vi "LVClass_WavefrontCorrector dtor.vi"(0 "WavefrontCorrector in":refnum<class "WavefrontCorrector.lvclass">, 11 "error in (no error)":errorcluster) -> (4 "WavefrontCorrector out":refnum<class "WavefrontCorrector.lvclass">, 15 "error out":errorcluster)   [LabVIEW 2020, in "WavefrontCorrector.lvclass"]
doc: "WavefrontCorrector destructor.\n\n--------------------------------------------------------------------------------\n\n<B>correctorIn </B> : WavefrontCorrector object.\n<B>correctorOut </B> : WavefrontCorrector object.\n<B>ErrorIn </B> : Error\n<B>ErrorOut </B> : Error\n\n--------------------------------------------------------------------------------"
uses:
  WavefrontCorrector.lvclass
  Controls/Wavefront Corrector states - ONE.ctl
  WavefrontCorrector.lvclass/WavefrontCorrector.ctl
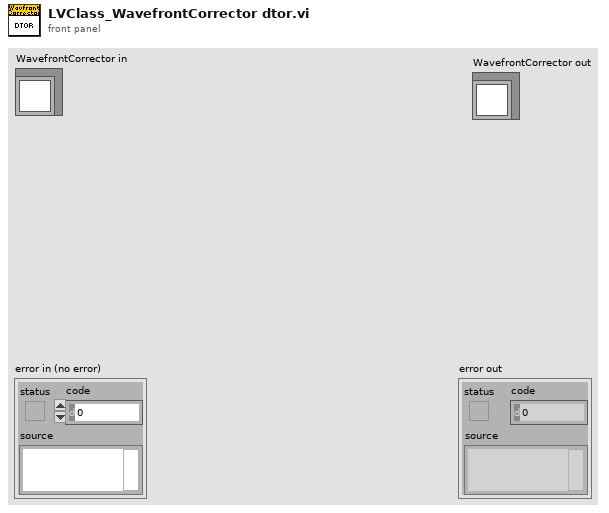
[diagram p1: front panel]
types:
  T1 = typedef "Wavefront Corrector states - ONE.ctl" = cluster{"Max":sgl, "Min":sgl, "Validity":enum16{"valid", "fixed", "invalid"}, "Fixed_Position":sgl}
  T2 = cluster{"Sleep after command apply_ms":i32, "Wavefront Corrector State":T1[]}
  T3 = typedef "Handle creation.ctl" = enum16{"By ctor", "By write function"}
  T4 = typedef "ClassID.ctl" = i64
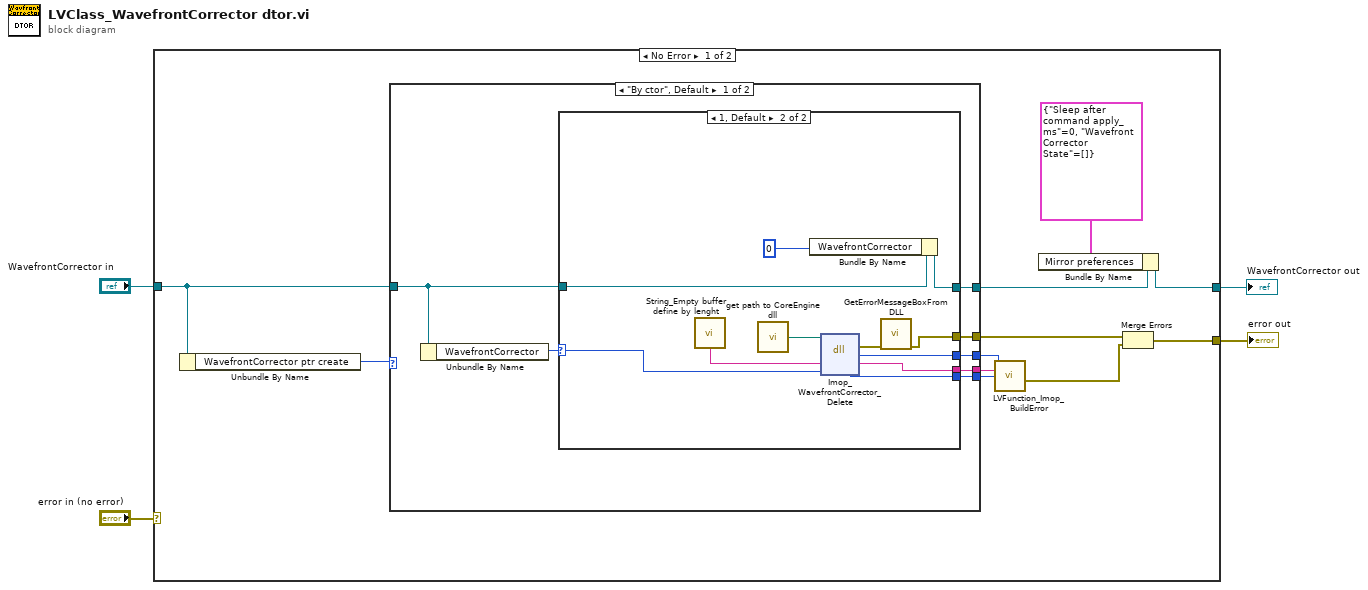
[diagram p0: block diagram]
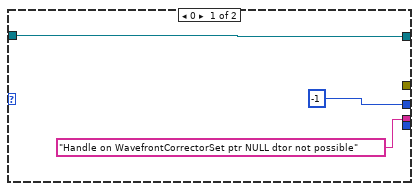
[diagram p2: hidden frame]
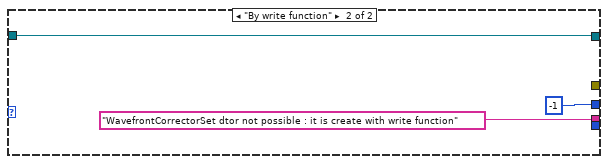
[diagram p3: hidden frame]
diagram:
  n1 = case shown="No Error" "error in (no error)" {
    selector: "error in (no error)" -> [_ w40]
    tunnel: "WavefrontCorrector in" -> [w13 w41]
    tunnel: [w7 w41] -> w1
    tunnel: [w9 w40] -> w2
    frame No Error {
      n2 = Unbundle By Name(w13) -> ("WavefrontCorrector ptr create"=w12:T3)
      n3 = case shown="\"By ctor\", Default" w12 {
        tunnel: [w22 "WavefrontCorrectorSet dtor not possible : it is create with write function" ("message")] -> w15
        tunnel: [w21 -1] -> w14
        tunnel: w13 -> [w19 w37]
        tunnel: [w20 w37] -> w8
        tunnel: [w17 _] -> w11
        tunnel: [w16 _] -> w5
        frame "By ctor", Default {
          n4 = Unbundle By Name(w19) -> ("WavefrontCorrector"=w18:T4)
          n5 = case shown="1, Default" w18 {
            selector: w18 -> [_ w33]
            tunnel: ["Handle on WavefrontCorrectorSet ptr NULL dtor not possible" ("message") w35] -> w22
            tunnel: [-1 w34] -> w21
            tunnel: w19 -> [w23 w29]
            tunnel: [w23 w28] -> w20
            tunnel: [_ w27] -> w17
            tunnel: [_ w26] -> w16
            frame 0 {
            }
            frame 1, Default {
              n6 = call "String_Empty buffer define by lenght.vi"() -> ("Empty buffer"=w36:string)  [unwired: 1 in]
              n7 = call "get path to CoreEngine dll.vi"() -> ("path to wavekit library"=w32:path)  [unwired: 14 in, 1 out]
              n8 = Bundle By Name(cluster=w29, "WavefrontCorrector"=u32 0 ("HasoEgine")) -> (w28:refnum<class "WavefrontCorrector.lvclass">)
              n9 = dll-call lib="D:/soft/HASO_v3/SVN_trunk/ImOpCoreEngine4_LV2011/DLLs/c_interface_vc100.dll" fn="Imop_WavefrontCorrector_Delete"(path in=w32, "message"=w36, "WavefrontCorrectionSet"=w33) -> (error out=w31:errorcluster, "return type"=w34:i32, "message"=w35:string, "WavefrontCorrectionSet"=w26:i64)  [unwired: 2 in, 1 out]
              n10 = call "GetErrorMessageBoxFromDLL.vi"("error IN"=w31) -> ("error OUT"=w27:errorcluster)  [unwired: 10 in]
            }
          }
        }
        frame "By write function" {
        }
      }
      n11 = call "LVFunction_Imop_BuildError.vi"("code"=w14, "String to Prepend to source (\"\")"=w15, "Adresse"=w5) -> ("error out"=w10:errorcluster)  [unwired: 12 in]
      n12 = Bundle By Name(cluster=w8, "Mirror preferences"=T2 {"Sleep after command apply_ms"=0, "Wavefront Corrector State"=[]}) -> (w7:refnum<class "WavefrontCorrector.lvclass">)
      n13 = Merge Errors(w11, w10) -> (w9:errorcluster)
    }
    frame Error {
    }
  }
  "error out" <- w2
  "WavefrontCorrector out" <- w1
